vi "WriteAppLog1.vi"(8 "error in (no error)":errorcluster, 11 "Msg":string) -> (0 "error out":errorcluster)   [LabVIEW 2024]
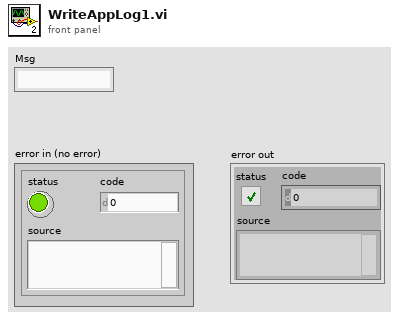
[diagram p1: front panel]
types:
  T1 = enum16{"open", "replace", "create", "open or create", "replace or create", "replace or create with confirmation"}
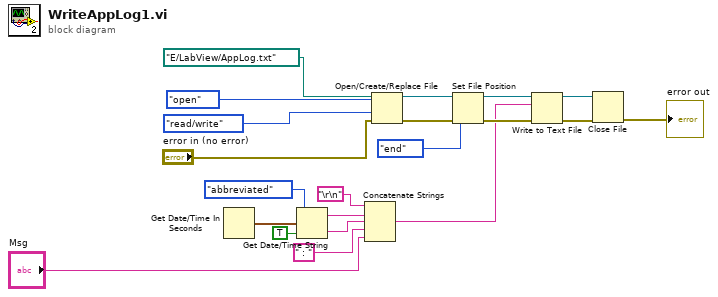
[diagram p0: block diagram]
diagram:
  n1 = Get Date/Time In Seconds() -> (seconds since 1Jan1904=w1:timestamp)
  n2 = Get Date/Time String(date format (0)=enum16{"short", "long", "abbreviated"}."abbreviated", seconds (now)=w1, want seconds? (F)=TRUE) -> (date string=w4:string, time string=w5:string)
  n3 = Concatenate Strings("\r\n", w4, w5, " : ", "Msg") -> (w16:string)
  n4 = Open/Create/Replace File(file path (use dialog)=path "E:/LabView/AppLog.txt", error in="error in (no error)", operation (0:open)=T1."open", access (0:read/write)=enum16{"read/write", "read-only", "write-only"}."read/write") -> (refnum out=w12:refnum<file>, error out=w14:errorcluster)  [unwired: 2 in, 1 out]
  n5 = Set File Position(refnum=w12, from (0:start)=enum16{"start", "end", "current"}."end", error in=w14) -> (refnum out=w15:refnum<file>, error out=w17:errorcluster)  [unwired: 1 in]
  n6 = Write to Text File(file (use dialog)=w15, text=w16, error in=w17) -> (refnum out=w18:refnum<file>, error out=w19:errorcluster)  [unwired: 1 in, 1 out]
  n7 = Close File(refnum=w18, error in=w19) -> (error out=→"error out":errorcluster)  [unwired: 1 out]
